vi "Get Position.vi"(8 "error in (no error)":errorcluster) -> (0 "error out":errorcluster, 2 "speeds":dbl[](array[numeric]), 3 "positions":dbl[](array[numeric]))   [LabVIEW 2020, in "Manipulator CLI Driver.lvlib"]
uses:
  Manipulator CLI Driver.lvlib
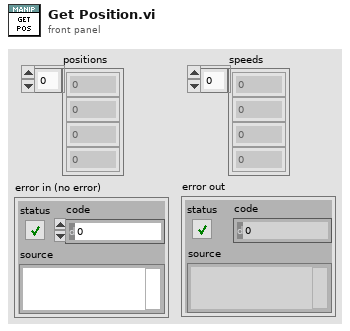
[diagram p1: front panel]
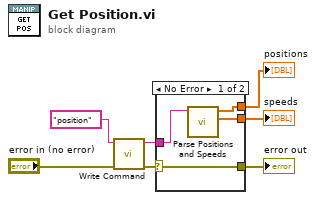
[diagram p0: block diagram]
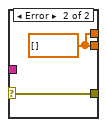
[diagram p2: hidden frame]
diagram:
  n1 = call "Write Command.vi"("error in (no error)"="error in (no error)", "command"="position") -> ("error out"=w5:errorcluster, "standard output"=w3:string)  [unwired: 7 in, 1 out]
  n2 = case shown="No Error" w5 {
    selector: w5 -> [w11 w13]
    tunnel: [w11 w13] -> w4
    tunnel: w3 -> [w10 _]
    tunnel: [w9 w12] -> w2
    tunnel: [w8 w12] -> w1
    frame No Error {
      n3 = call "Parse Positions and Speeds.vi"("standard output"=w10) -> ("Array"=w8:dbl[], "Array 2"=w9:dbl[])  [unwired: 9 in]
    }
    frame Error {
      w12 = dbl[] []
    }
  }
  "error out" <- w4
  "positions" <- w2
  "speeds" <- w1
